vi "Read target.vi"(8 "error in (no error)":errorcluster, 11 "Client_s4gui in":refnum<class "Client_s4gui.lvclass">) -> (0 "error out":errorcluster, 2 "target":dbl, 3 "Client_s4gui out":refnum<class "Client_s4gui.lvclass">)   [LabVIEW 2018, in "Client_s4gui.lvclass"]
uses:
  Client_s4gui.lvclass
  Client_s4gui.lvclass/Client_s4gui.ctl
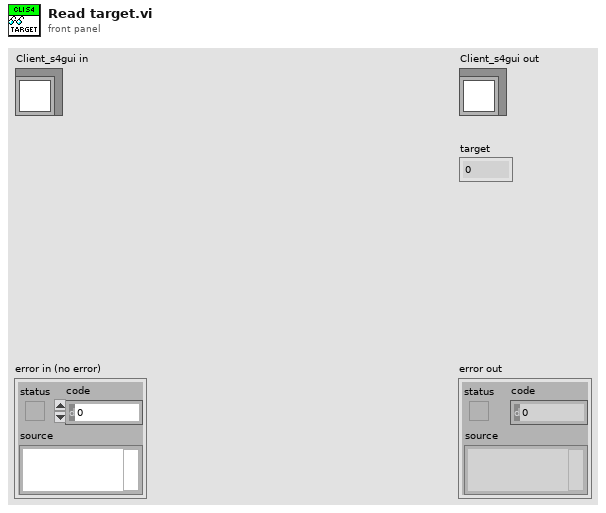
[diagram p1: front panel]
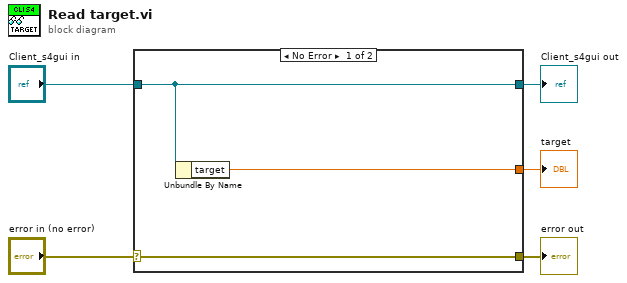
[diagram p0: block diagram]
diagram:
  n1 = case shown="No Error" "error in (no error)" {
    selector: "error in (no error)" -> [w8 w9]
    tunnel: [w8 w9] -> w4
    tunnel: [w7 w10] -> w2
    tunnel: "Client_s4gui in" -> [w7 w10]
    tunnel: [w6 _] -> w1
    frame No Error {
      n2 = Unbundle By Name(w7) -> ("target"=w6:dbl)
    }
    frame Error {
    }
  }
  "error out" <- w4
  "Client_s4gui out" <- w2
  "target" <- w1
